vi "save live config to db.vi"(6 "configuration name":string, 7 "experiment name":string, 8 "error in (no error)":errorcluster, 9 "Device Name":string, 10 "variable values":string[](array[string]), 11 "Variable names (inc device)":string[](array[string])) -> (0 "error out":errorcluster)   [LabVIEW 2020]
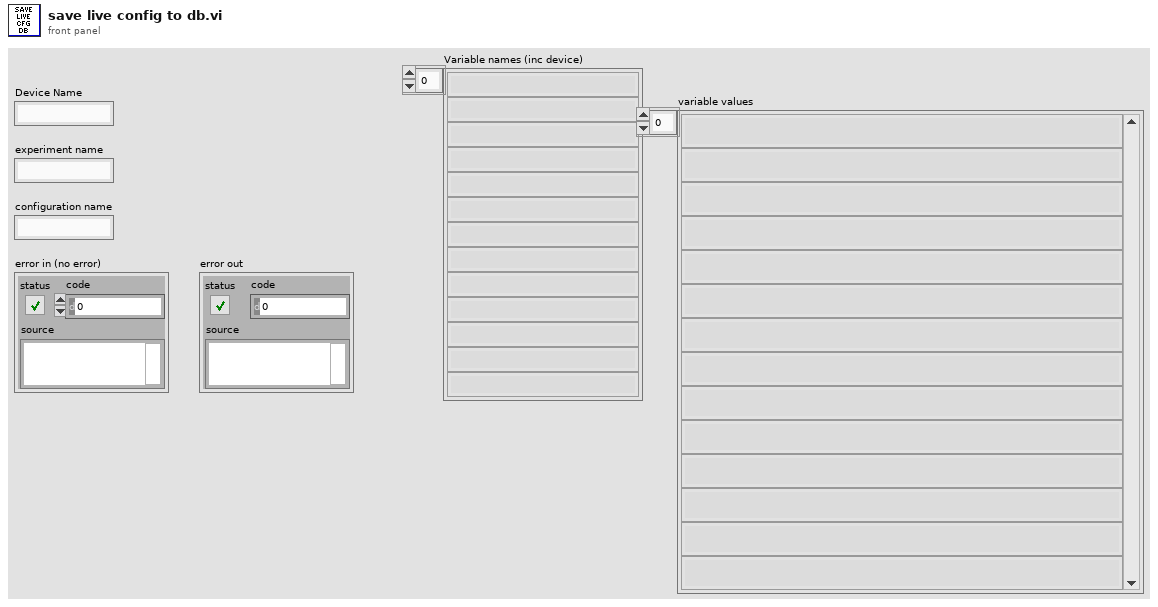
[diagram p1: front panel]
types:
  T1 = typedef "mysql_authentication.ctl" = cluster{"User":string, "Password":string, "Database":string}
  T2 = cluster{"Port":u16, "IP Address":string, "Authentication":T1}
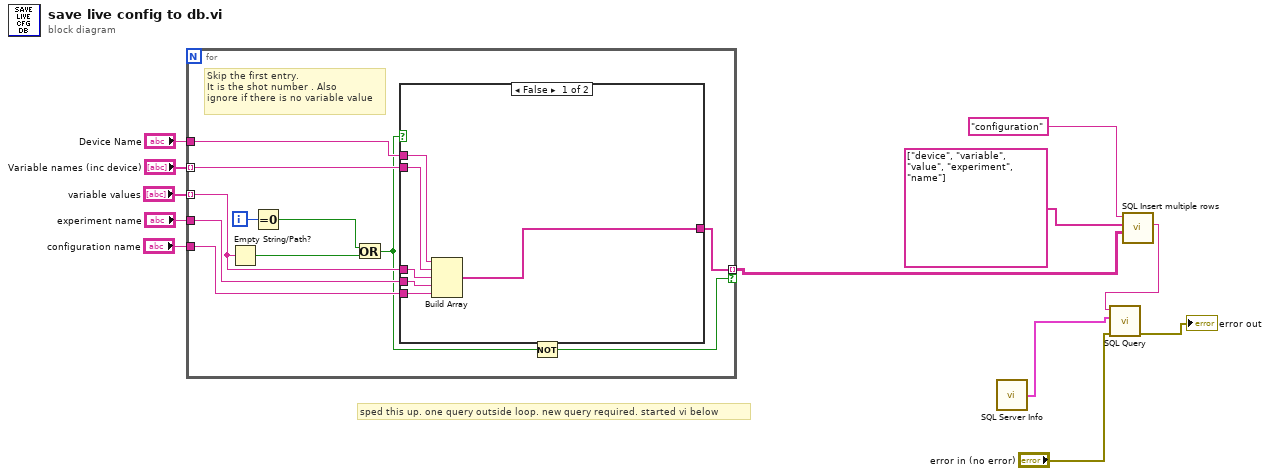
[diagram p0: block diagram]
diagram:
  # "sped this up. one query outside loop. new query required. started vi below"
  n1 = for {
    tunnel: "configuration name" -> [w23]
    tunnel: "experiment name" -> [w22]
    tunnel: "Device Name" -> [w21]
    tunnel: "Variable names (inc device)" -> [w20] mode=indexing
    tunnel: "variable values" -> [w17] mode=indexing
    tunnel: [w14] -> w5 mode=indexing if=w13
    i -> [w19]
    # "Skip the first entry.\nIt is the shot number . Also\nignore if there is no variable value"
    n2 = Empty String/Path?(string/path=w17) -> (empty?=w16:bool)
    n3 = Equal To 0?(x=w19) -> (x = 0?=w18:bool)
    n4 = Or(x=w18, y=w16) -> (x .or. y?=w15:bool)
    n5 = case shown="False" w15 {
      tunnel: w23 -> [w29 _]
      tunnel: w22 -> [w28 _]
      tunnel: w21 -> [w27 _]
      tunnel: w20 -> [w26 _]
      tunnel: w17 -> [w25 _]
      tunnel: [w24 _] -> w14
      frame False {
        n6 = Build Array(w27, w26, w25, w28, w29) -> (w24:string[])
      }
      frame True {
      }
    }
    n7 = Not(x=w15) -> (.not. x?=w13:bool)
  }
  n8 = call "SQL Server Info.vi"() -> ("SQL Server Info"=w4:T2)
  n9 = call "SQL Insert multiple rows.vi"("Values"=w5, "Column Names"=string[] ["device", "variable", "value", "experiment", "name"], "Table"="configuration") -> ("Query String"=w2:string)  [unwired: 8 in]
  n10 = call "SQL Query.vi"("error in (no error)"="error in (no error)", "SQL Server Info"=w4, "Query"=w2) -> ("error out"=→"error out":errorcluster)  [unwired: 7 in, 1 out]
